vi "TSM Get Functional Test Settings.vi"(0 "TSM context":T2, 11 "error in (no error)":errorcluster) -> (2 "Coarse Freq Sweep (Hz)":T1 {"End" format="%#_13g"; "Start" format="%#_13g"}, 3 "Fine Freq Sweep (Hz)":T1 {"End" format="%#_13g"; "Start" format="%#_13g"}, 4 "TSM context Out":T2, 6 "Limit (dB SPL)":dbl, 8 "Speaker Amplitude (V)":dbl, 15 "error out":errorcluster)   [LabVIEW 2020]
doc: "Get the DAQmx Analog Output settings of the Speaker from the spec sheet using TSM context"
uses:
  <vilib>/NI_TestStand_SemiconductorModule/NI_TestStand_Semiconductor_Module.lvlibp/PinMap/General/SemiconductorModuleContext.ctl
  Utility/Calibration Sweep/Sweep Parameters.ctl
  <vilib>/NI_TestStand_SemiconductorModule/NI_TestStand_Semiconductor_Module.lvlibp/PinMap/Specs/NamespacedSymbolsToValues.vi
  <vilib>/NI_TestStand_SemiconductorModule/NI_TestStand_Semiconductor_Module.lvlibp
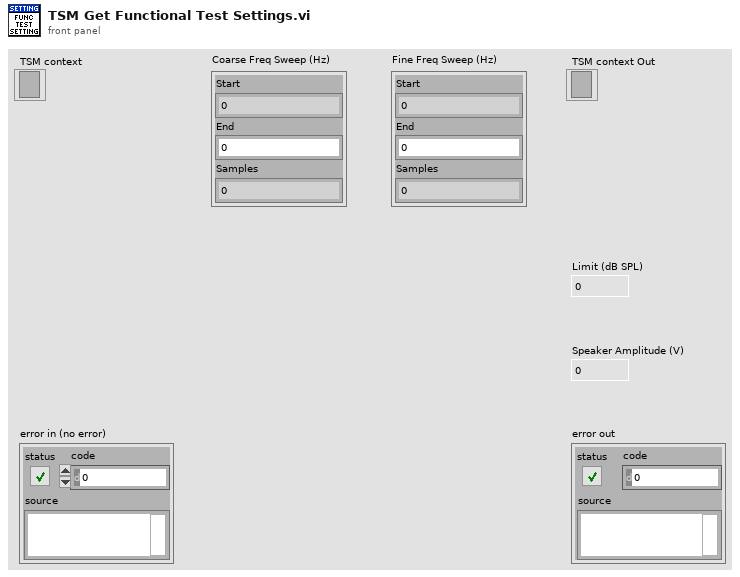
[diagram p1: front panel]
types:
  T1 = typedef "Sweep Parameters.ctl" = cluster{"Start":dbl, "End":dbl, "Samples":i32}
  T2 = typedef "NI_TestStand_Semiconductor_Module.lvlibp/SemiconductorModuleContext.ctl" = refnum<k7>
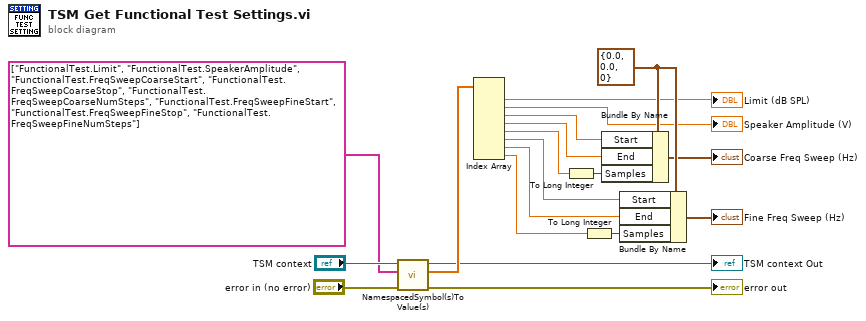
[diagram p0: block diagram]
diagram:
  w11 = T1 {"Start"=0.0, "End"=0.0, "Samples"=0} ("Sweep Parameters")
  n1 = call-poly <vilib>:"NamespacedSymbol(s)ToValue(s).vi"("error in (no error)"="error in (no error)", "Symbols"=tag[] ["FunctionalTest.Limit", "FunctionalTest.SpeakerAmplitude", "FunctionalTest.FreqSweepCoarseStart", "FunctionalTest.FreqSweepCoarseStop", "FunctionalTest.FreqSweepCoarseNumSteps", "FunctionalTest.FreqSweepFineStart", "FunctionalTest.FreqSweepFineStop", "FunctionalTest.FreqSweepFineNumSteps"], "Semiconductor Module Context"="TSM context") -> ("error out"=→"error out":errorcluster, "Values"=w16:dbl[], "Semiconductor Module Context Out"=→"TSM context Out":T2)  [unwired: 6 in]
  n2 = Index Array(array=w16) -> (element #1=→"Limit (dB SPL)":dbl, element #2=→"Speaker Amplitude (V)":dbl, element #3=w6:dbl, element #4=w5:dbl, element #5=w4:dbl, element #6=w3:dbl, element #7=w2:dbl, element #8=w1:dbl)  [unwired: 8 in]
  n3 = To Long Integer(number=w4) -> (32bit integer=w13:i32)
  n4 = To Long Integer(number=w1) -> (32bit integer=w12:i32)
  n5 = Bundle By Name(cluster=w11, "Start"=w6, "End"=w5, "Samples"=w13) -> (→"Coarse Freq Sweep (Hz)":T1)
  n6 = Bundle By Name(cluster=w11, "Start"=w3, "End"=w2, "Samples"=w12) -> (→"Fine Freq Sweep (Hz)":T1)
